vi "TitlePage.vi"(2 "Graph":T1={"GraphCtl Refnum"=refnum, "Wrap Text (F:No)"=FALSE, "Hide Grid (F:No)"=FALSE, "Scale (100%)"=100.0, "Align (Left)"=0, "PositionBemerkung"=enum."before", "PageBreak"=enum."before"} {"Align (Left)" items=["Center", "Justified", "Justified All", "Left", "Right"]}, 4 "TableFont":T5[](array[typedef]), 5 "HeaderTableFonts":T5[](array[typedef]), 6 "Title Font":T5={"Font"="Arial", "Size"=26, "Colour"=0, "Bold"=TRUE, "Italic"=FALSE, "Underline"=TRUE, "Strikethrough"=FALSE, "Font Encoding"=enum."Cp1252, WinANSI"}, 7 "Column Ratios left":sgl[][](array[numeric]), 8 "error in":errorcluster, 9 "Table Array":T7[](array[typedef]) {"Horizontal Align" items=["Center", "Justified", "JustifiedAll", "Left", "Right"]; "TablePictures"."Horizontal Align" items=["Center", "Justified", "JustifiedAll", "Left", "Right"]; "Results"."Position" items=["First", "Last"]; "Results"."Horizontal Align" items=["Center", "Justified", "JustifiedAll", "Left", "Right"]}, 10 "Content":T11={"Titel"="Test mit Graph PDF", "Header Tables"=[[["Murks:", "4711"], ["HolyShit:", "0815"]]], "Bemerkungen"=[]} {"Bemerkungen"."Align (Left)" items=["Center", "Justified", "Justified All", "Left", "Right"]}, 11 "Context (Eingang)":refnum<class "Context.lvclass">) -> (0 "error out":errorcluster, 3 "Context (Ausgang)":refnum<class "Context.lvclass">)   [LabVIEW 2020, in "PDF Interface.lvlib"]
doc: "To add Content to a PDF Page that was created by \"InitBeforePage\" or after \"AddAdditionalPage\"."
uses:
  PDF Interface.lvlib
  <vilib>/Simplicity AI/SAI_PDF_API/Classes/Context/Controls/SAI_PDF_Font.ctl
  <vilib>/Simplicity AI/SAI_PDF_API/Classes/Context/Controls/SAI_PDF_Font Encoding.ctl
  PDF Interface Helper/PDFTtilePageContentType.ctl
  PDF Interface Helper/PDFBemerkung.ctl
  <vilib>/Simplicity AI/SAI_PDF_API/Classes/Context/Controls/SAI_PDF_Text Align.ctl
  <vilib>/Simplicity AI/SAI_PDF_API/Classes/Context/Context.lvclass
  PDF Interface Helper/PDFTableContentType.ctl
  PDF Interface Helper/PDFResults.ctl
  PDF Interface Helper/PDFResultPictures.ctl
  PDF Interface Helper/PDFCommentPosition.ctl
  PDF Interface Helper/PDFPageBreak.ctl
  PDF Interface Helper/PDFTablePictures.ctl
  PDF Interface Helper/PDFGraph.ctl
  PDF Interface Helper/PDF Interface Helper.lvlib
panel:
  # "(Cp1252)"
  # "(Cp1252)"
  # "(Cp1252)"
  # "(Cp1252)"
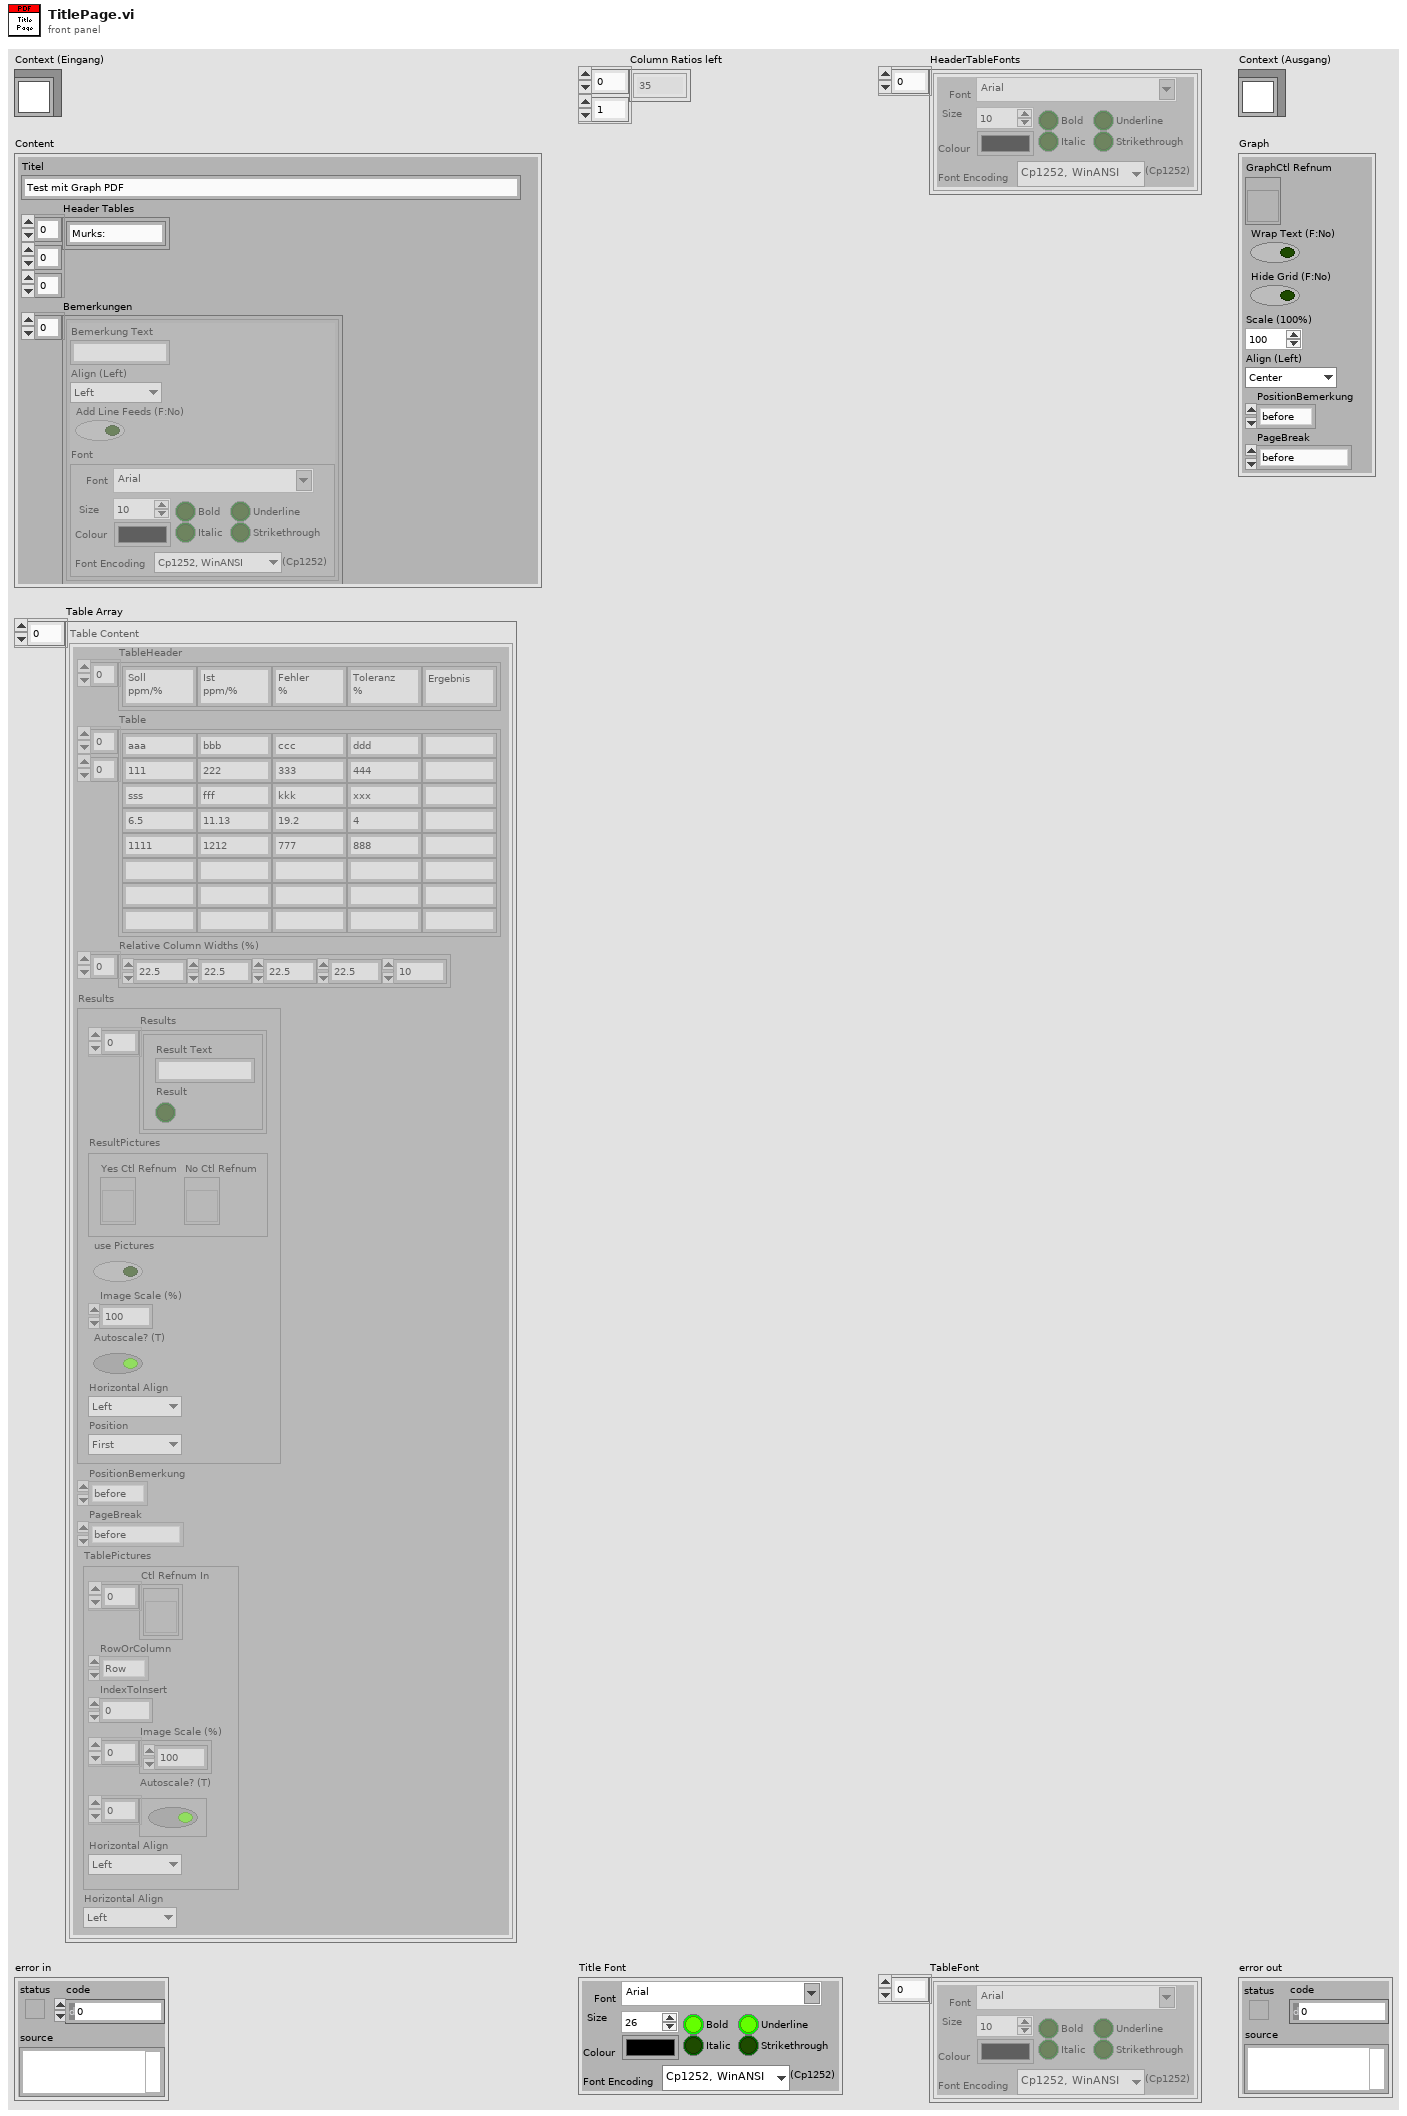
[diagram p1: front panel]
types:
  T1 = typedef "PDF Interface.lvlib/PDF Interface Helper.lvlib/PDFGraph.ctl" = cluster{"GraphCtl Refnum":refnum<vi>, "Wrap Text (F:No)":bool, "Hide Grid (F:No)":bool, "Scale (100%)":sgl, "Align (Left)":T2, "PositionBemerkung":T3, "PageBreak":T4}
  T2 = typedef "SAI_PDF_Toolkit.lvlib/Context.lvclass/SAI_PDF_Text Align.ctl" = i32
  T3 = typedef "PDF Interface.lvlib/PDF Interface Helper.lvlib/PDFCommentPosition.ctl" = enum16{"before", "after"}
  T4 = typedef "PDF Interface.lvlib/PDF Interface Helper.lvlib/PDFPageBreak.ctl" = enum16{"none", "before", "after", "after comment"}
  T5 = typedef "SAI_PDF_Toolkit.lvlib/Context.lvclass/SAI_PDF_Font.ctl" = cluster{"Font":string, "Size":i32, "Colour":u32, "Bold":bool, "Italic":bool, "Underline":bool, "Strikethrough":bool, "Font Encoding":T6}
  T6 = typedef "SAI_PDF_Toolkit.lvlib/Context.lvclass/SAI_PDF_Font Encoding.ctl" = enum16{"Cp1252, WinANSI", "IdentityH", "IdentityV", "Cp1250", "Cp1257", "MacRoman"}
  T7 = typedef "PDF Interface.lvlib/PDF Interface Helper.lvlib/PDFTableContentType.ctl" = cluster{"TableHeader":string[], "Table":string[][], "Relative Column Widths (%)":sgl[], "Results":T8, "PositionBemerkung":T3, "PageBreak":T4, "TablePictures":T10, "Horizontal Align":i32}
  T8 = typedef "PDF Interface.lvlib/PDF Interface Helper.lvlib/PDFResults.ctl" = cluster{"Results":cluster{"Result Text":string, "Result":bool}[], "ResultPictures":T9, "use Pictures":bool, "Image Scale (%)":sgl, "Autoscale? (T)":bool, "Horizontal Align":i32, "Position":i32}
  T9 = typedef "PDF Interface.lvlib/PDF Interface Helper.lvlib/PDFResultPictures.ctl" = cluster{"Yes Ctl Refnum":refnum<vi>, "No Ctl Refnum":refnum<vi>}
  T10 = typedef "PDF Interface.lvlib/PDF Interface Helper.lvlib/PDFTablePictures.ctl" = cluster{"Ctl Refnum In":refnum<vi>[], "RowOrColumn":enum16{"Row", "Column"}, "IndexToInsert":u16, "Image Scale (%)":sgl[], "Autoscale? (T)":bool[], "Horizontal Align":i32}
  T11 = typedef "PDF Interface.lvlib/PDF Interface Helper.lvlib/PDFTtilePageContentType.ctl" = cluster{"Titel":string, "Header Tables":string[][][], "Bemerkungen":T12[]}
  T12 = typedef "PDF Interface.lvlib/PDF Interface Helper.lvlib/PDFBemerkung.ctl" = cluster{"Bemerkung Text":string, "Align (Left)":T2, "Add Line Feeds (F:No)":bool, "Font":T5}
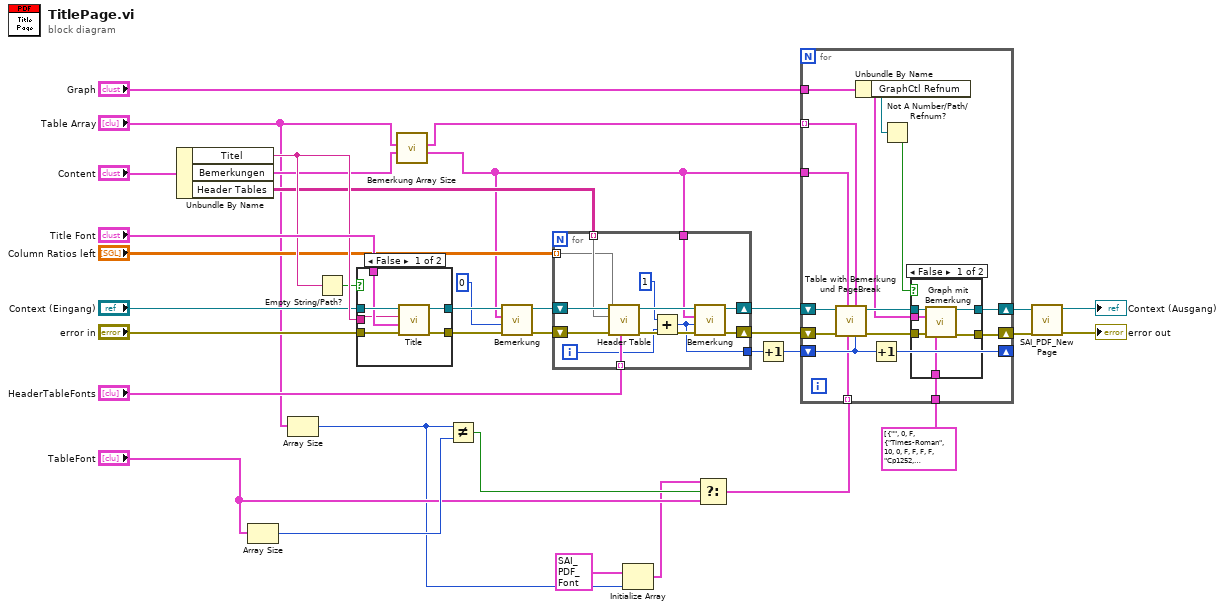
[diagram p0: block diagram]
diagram:
  n1 = Unbundle By Name("Content") -> ("Titel"=w27:string, "Bemerkungen"=w12:T12[], "Header Tables"=w25:string[][][])
  n2 = Array Size(array="TableFont") -> (size(s)=w9:i32)
  n3 = Array Size(array="Table Array") -> (size(s)=w3:i32)
  n4 = Empty String/Path?(string/path=w27) -> (empty?=w26:bool)
  n5 = case shown="False" w26 {
    tunnel: [w41 w43] -> w35
    tunnel: [w40 w42] -> w34
    tunnel: "error in" -> [w39 w42]
    tunnel: "Context (Eingang)" -> [w38 w43]
    tunnel: "Title Font" -> [w37 _]
    tunnel: w27 -> [w36 _]
    frame False {
      n6 = call "Title.vi"("error in (no error)"=w39, "Font"=w37, "Text"=w36, "Context in"=w38) -> ("error out"=w40:errorcluster, "Context out"=w41:refnum<class "Context.lvclass">)  [unwired: 3 in, 3 out]
    }
    frame True {
    }
  }
  n7 = call "Bemerkung Array Size.vi"("Bemerkungen (Eingang)"=w12, "Table Array (Eingang)"="Table Array") -> ("Bemerkungen (Ausgang)"=w11:T12[], "Table Array (Ausgang)"=w13:T7[])  [unwired: 6 in, 2 out]
  n8 = Not Equal?(x=w3, y=w9) -> (x != y?=w8:bool)
  n9 = call "Bemerkung.vi"("Fehler (Eingang, kein Fehler)"=w34, "Index"=0, "Bemerkung"=w11, "Context (Eingang)"=w35) -> ("Fehler (Ausgang)"=w32:errorcluster, "Context (Ausgang)"=w33:refnum<class "Context.lvclass">)  [unwired: 6 in]
  n10 = for {
    tunnel: w11 -> [w51]
    tunnel: w25 -> [w50] mode=indexing
    tunnel: "Column Ratios left" -> [w49] mode=indexing
    tunnel: "HeaderTableFonts" -> [w48] mode=indexing
    shift-right: [w47] -> w19
    shift-left: w33 -> [w56]
    shift-right: [w46] -> w17
    shift-left: w32 -> [w55]
    tunnel: [w44] -> w15
    i -> [w45]
    n11 = call "Header Table.vi"("Font"=w48, "error in"=w55, "Column Ratio left"=w49, "Table"=w50, "Context In"=w56) -> ("error out"=w53:errorcluster, "Context Out"=w54:refnum<class "Context.lvclass">)  [unwired: 5 in]
    n12 = Add(x=1 ("Index"), y=w45) -> (x+y=w44:i32)
    n13 = call "Bemerkung.vi"("Fehler (Eingang, kein Fehler)"=w53, "Index"=w44, "Bemerkung"=w51, "Context (Eingang)"=w54) -> ("Fehler (Ausgang)"=w46:errorcluster, "Context (Ausgang)"=w47:refnum<class "Context.lvclass">)  [unwired: 6 in]
  }
  n14 = Initialize Array(T5 {"Font"="Arial", "Size"=10, "Colour"=0, "Bold"=FALSE, "Italic"=FALSE, "Underline"=FALSE, "Strikethrough"=FALSE, "Font Encoding"=enum."Cp1252, WinANSI"} ("TableFont"), w3) -> (w5:T5[])
  n15 = Select(t=w5, s=w8, f="TableFont") -> (s? t:f=w4:T5[])
  n16 = Increment(x=w15) -> (x+1=w14:i32)
  n17 = for {
    tunnel: w11 -> [w69]
    tunnel: w13 -> [w68] mode=indexing
    shift-right: [w61] -> w18
    shift-left: w19 -> [w71]
    shift-right: [w63] -> w16
    shift-left: w17 -> [w70]
    shift-right: [w66] -> _
    shift-left: w14 -> [w67]
    tunnel: w4 -> [w65] mode=indexing
    tunnel: "Graph" -> [w59]
    tunnel: T12[] [{"Bemerkung Text"="", "Align (Left)"=0, "Add Line Feeds (F:No)"=FALSE, "Font"={"Font"="Times-Roman", "Size"=10, "Colour"=0, "Bold"=FALSE, "Italic"=FALSE, "Underline"=FALSE, "Strikethrough"=FALSE, "Font Encoding"=enum."Cp1252, WinANSI"}}] ("Bemerkungen") -> [w60]
    n18 = call "Table with Bemerkung und PageBreak.vi"("Index"=w67, "Table Content"=w68, "TableFont"=w65, "Bemerkungen"=w69, "Fehler (Eingang, kein Fehler)"=w70, "Context (Eingang)"=w71) -> ("Fehler (Ausgang)"=w64:errorcluster, "Context (Ausgang)"=w62:refnum<class "Context.lvclass">)  [unwired: 4 in]
    n19 = Unbundle By Name(w59) -> ("GraphCtl Refnum"=w58:refnum<vi>)
    n20 = Increment(x=w67) -> (x+1=w66:i32)
    n21 = Not A Number/Path/Refnum?(number/path/refnum=w58) -> (NaN/Path/Refnum?=w57:bool)
    n22 = case shown="False" w57 {
      tunnel: w59 -> [w77 _]
      tunnel: w64 -> [w76 w78]
      tunnel: [w75 w78] -> w63
      tunnel: w62 -> [w74 w79]
      tunnel: [w73 w79] -> w61
      tunnel: w60 -> [w72 _]
      frame False {
        n23 = call "Graph mit Bemerkung.vi"("Context (Eingang)"=w74, "Graph"=w77, "Fehler (Eingang, kein Fehler)"=w76, "Bemerkungen"=w72) -> ("Context (Ausgang)"=w73:refnum<class "Context.lvclass">, "Fehler (Ausgang)"=w75:errorcluster)  [unwired: 9 in, 1 out]
      }
      frame True {
      }
    }
  }
  n24 = call <vilib>:"SAI_PDF_New Page.vi"("error in"=w16, "Context In"=w18) -> ("error out"=→"error out":errorcluster, "Context Out"=→"Context (Ausgang)":refnum<class "Context.lvclass">)  [unwired: 8 in]
